vi "Bar Graph.vi"() -> ()   [LabVIEW 2016]
panel:
  out "Beta":dbl(slide) scale=0.0..100.0
  out "Alpha":dbl(slide) scale=0.0..100.0
  out "Theta":dbl(slide) scale=0.0..100.0
  # "Theta"
  # "Alpha"
  # "Beta"
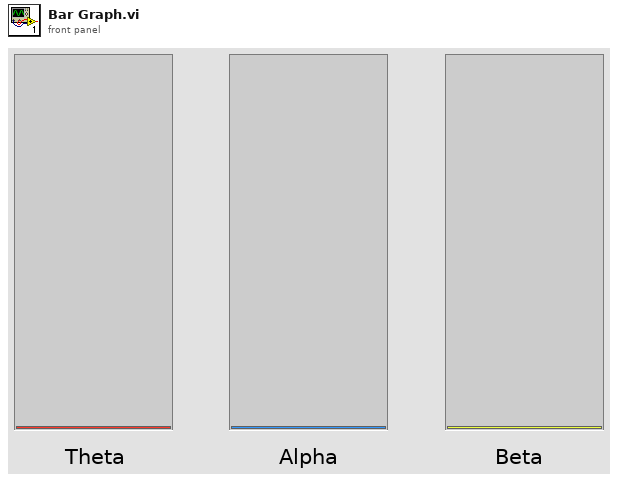
[diagram p1: front panel]
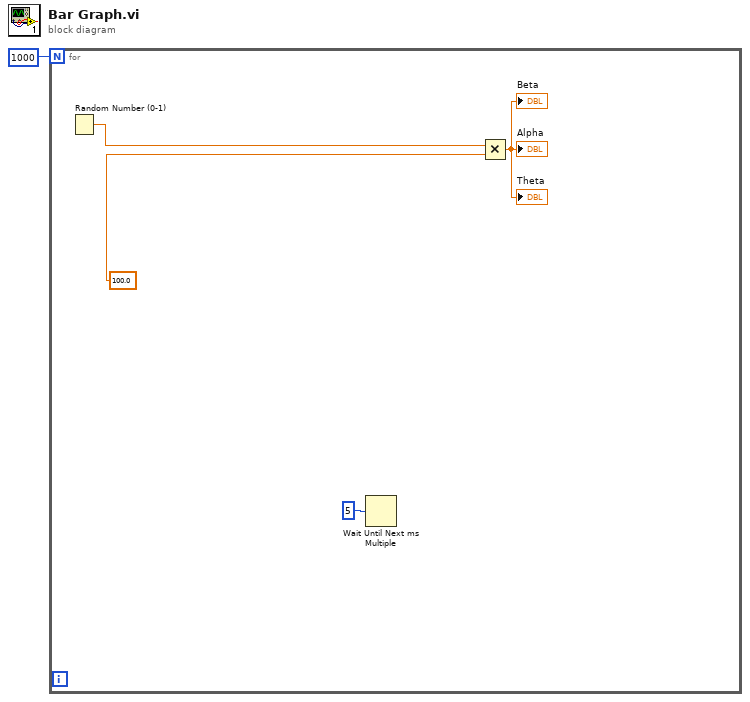
[diagram p0: block diagram]
diagram:
  n1 = for {
    N: 1000 -> [_]
    n2 = Random Number (0-1)() -> (number: 0 to 1=w4:dbl)
    n3 = Wait Until Next ms Multiple(millisecond multiple=u32 5) -> ()  [unwired: 1 out]
    n4 = Multiply(x=w4, y=100.0) -> (x*y=→"Theta" →"Alpha" →"Beta":dbl)
  }
